vi "ReadCSV_LogFiles.vi"() -> (3 "all rows 2":string[][](array[string]))   [LabVIEW 2018, in "RW_Protocols.lvlib"]
uses:
  RW_Protocols.lvlib
  <vilib>/Utility/file.llb/Read Delimited Spreadsheet (string).vi
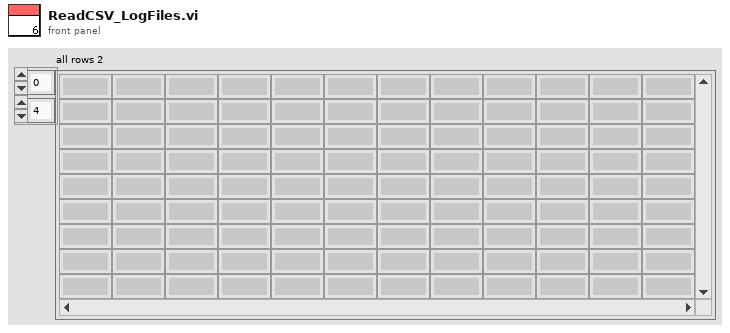
[diagram p1: front panel]
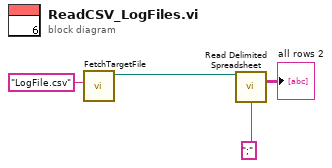
[diagram p0: block diagram]
diagram:
  n1 = call "FetchTargetFile.vi"("FileName"="LogFile.csv") -> ("Full File Path"=w3:path)  [unwired: 10 in]
  n2 = call-poly <vilib>:"Read Delimited Spreadsheet.vi"("file path (dialog if empty)"=w3, "delimiter (\\t)"=";" ("delimiter (\\t)")) -> ("all rows"=→"all rows 2":string[][])  [unwired: 8 in, 5 out]
